vi "4G Write.vi"(3 "error in (no error)":errorcluster, 4 "write buffer (\"\")":string, 5 "VISA session":refnum<visa-resource-name>) -> (0 "error out":errorcluster, 1 "return count":u32, 2 "dup VISA session":refnum<visa-resource-name>)   [LabVIEW 2010]
doc: "CS-4 Write.vi sends a command to to the CS-4 using a VISA channel previously opened by CS-4 Initialize.vi. \n\nIf a serial interface is used the input buffer is flushed by discarding the available bytes. It also verifies and strips command echo from\nthe input buffer. If a valid echo is not received on a serial channel a VISA READ timeout will occur."
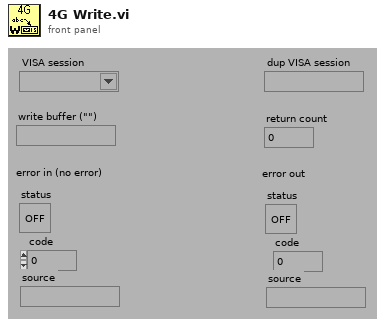
[diagram p1: front panel]
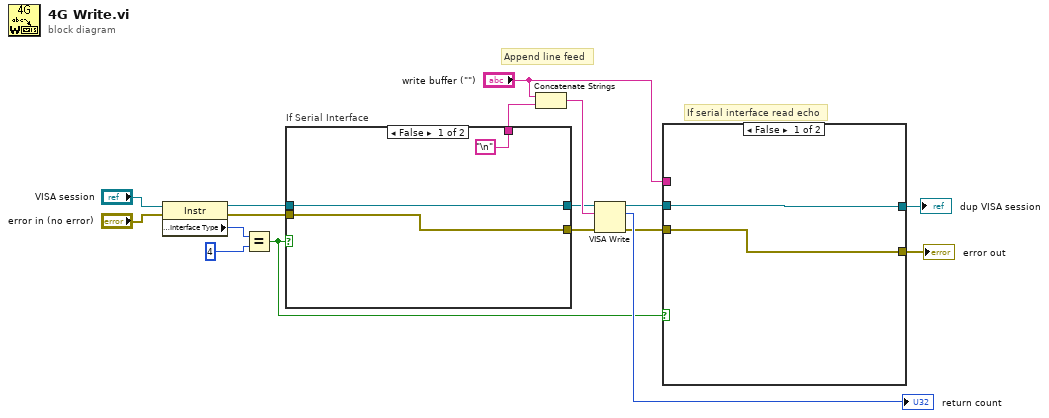
[diagram p0: block diagram]
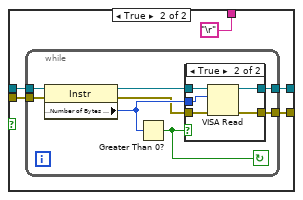
[diagram p2: hidden frame]
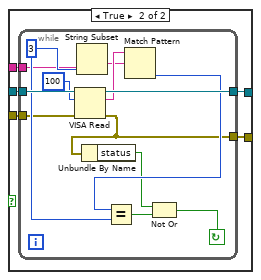
[diagram p4: hidden frame]
diagram:
  # "Append line feed"
  # "If serial interface read echo"
  n1 = property class="Instr"(reference="VISA session", error in="error in (no error)") -> (reference out=w4:refnum<visa-resource-name>, error out=w5:errorcluster, "Interface Information:Interface Type"=w2:u16)
  n2 = Equal?(x=w2, y=u16 4) -> (x = y?=w1:bool)
  n3 = case "If Serial Interface" shown="False" w1 {
    tunnel: [w20 w22] -> w7
    tunnel: [w19 w23] -> w6
    tunnel: w5 -> [w19 w25]
    tunnel: w4 -> [w20 w24]
    tunnel: ["\n" "\r"] -> w3
    frame False {
    }
    frame True {
      n4 = while {
        tunnel: w25 -> [w28]
        tunnel: w24 -> [w29]
        tunnel: [w32] -> w23
        tunnel: [w33] -> w22
        stop <- w26 continue-if-true
        n5 = property class="Instr"(reference=w29, error in=w28) -> (reference out=w30:refnum<visa-resource-name>, error out=w27:errorcluster, "Serial Settings:Number of Bytes at Serial Port"=w31:u32)
        n6 = Greater Than 0?(x=w31) -> (x > 0?=w26:bool)
        n7 = case shown="True" w26 {
          tunnel: w31 -> [_ w40]
          tunnel: w27 -> [w34 w39]
          tunnel: w30 -> [w35 w38]
          tunnel: [w34 w37] -> w32
          tunnel: [w35 w36] -> w33
          frame False {
          }
          frame True {
            n8 = VISA Read(VISA resource name=w38, byte count=w40, error in (no error)=w39) -> (VISA resource name out=w36:refnum<visa-resource-name>, error out=w37:errorcluster)  [unwired: 2 out]
          }
        }
      }
    }
  }
  n9 = Concatenate Strings("write buffer (\"\")", w3) -> (w13:string)
  n10 = VISA Write(VISA resource name=w7, write buffer=w13, error in (no error)=w6) -> (VISA resource name out=w8:refnum<visa-resource-name>, return count=→"return count":u32, error out=w9:errorcluster)
  n11 = case shown="False" w1 {
    tunnel: w8 -> [w42 w46]
    tunnel: w9 -> [w41 w47]
    tunnel: [w42 w45] -> w16
    tunnel: [w41 w43] -> w15
    tunnel: "write buffer (\"\")" -> [_ w44]
    frame False {
    }
    frame True {
      n12 = while {
        tunnel: [w51] -> w43
        tunnel: w44 -> [w48]
        tunnel: w47 -> [w52]
        tunnel: w46 -> [w59]
        tunnel: [w60] -> w45
        stop <- w56 continue-if-true
        w55 = 3 ("length")
        n13 = VISA Read(VISA resource name=w59, byte count=u32 100 ("byte count (0)"), error in (no error)=w52) -> (VISA resource name out=w60:refnum<visa-resource-name>, read buffer=w57:string, error out=w51:errorcluster)  [unwired: 1 out]
        n14 = String Subset(string=w48, length (rest)=w55) -> (substring=w54:string)  [unwired: 1 in]
        n15 = Unbundle By Name(w51) -> ("status"=w49:bool)
        n16 = Match Pattern(string=w57, regular expression=w54) -> (offset past match=w53:i32)  [unwired: 1 in, 3 out]
        n17 = Equal?(x=w53, y=w55) -> (x = y?=w50:bool)
        n18 = Not Or(1:w50, 2:w49) -> (0:w56:bool)
      }
    }
  }
  "dup VISA session" <- w16
  "error out" <- w15
